vi "All the different Gates.vi"() -> ()   [LabVIEW 2021]
panel:
  out "Boolean 3":bool
  in  "Boolean 2":bool
  in  "Boolean":bool
  out "LED(Output) 6":bool
  in  "B 6":bool
  in  "A 6":bool
  out "LED(Output) 5":bool
  in  "B 5":bool
  in  "A 5":bool
  out "LED(Output) 4":bool
  in  "B 4":bool
  in  "A 4":bool
  out "LED(Output) 3":bool
  in  "B 3":bool
  in  "A 3":bool
  out "LED(Output) 2":bool
  in  "A 2":bool
  out "LED(Output)":bool
  in  "B":bool
  in  "A":bool
  out "LED(Output)":bool
  in  "B":bool
  in  "A":bool
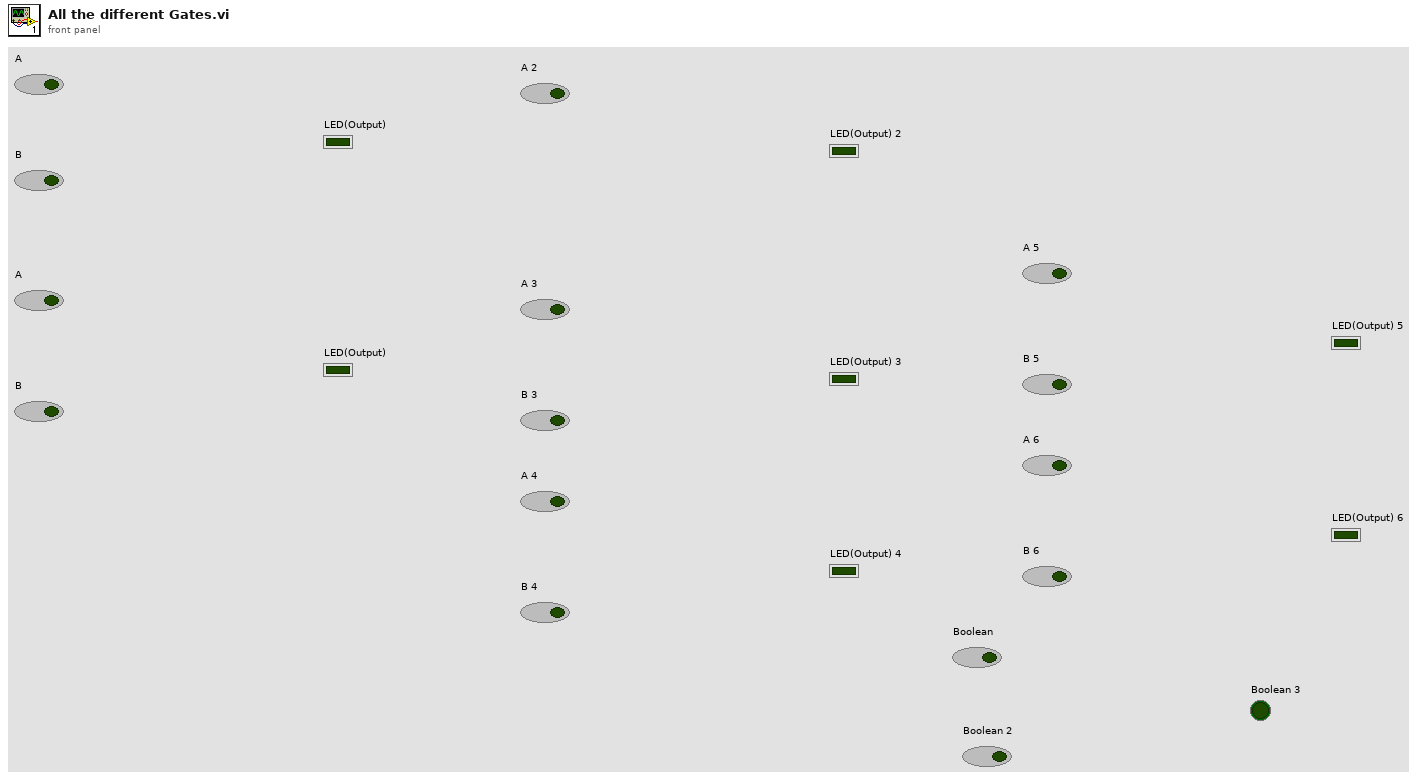
[diagram p1: front panel]
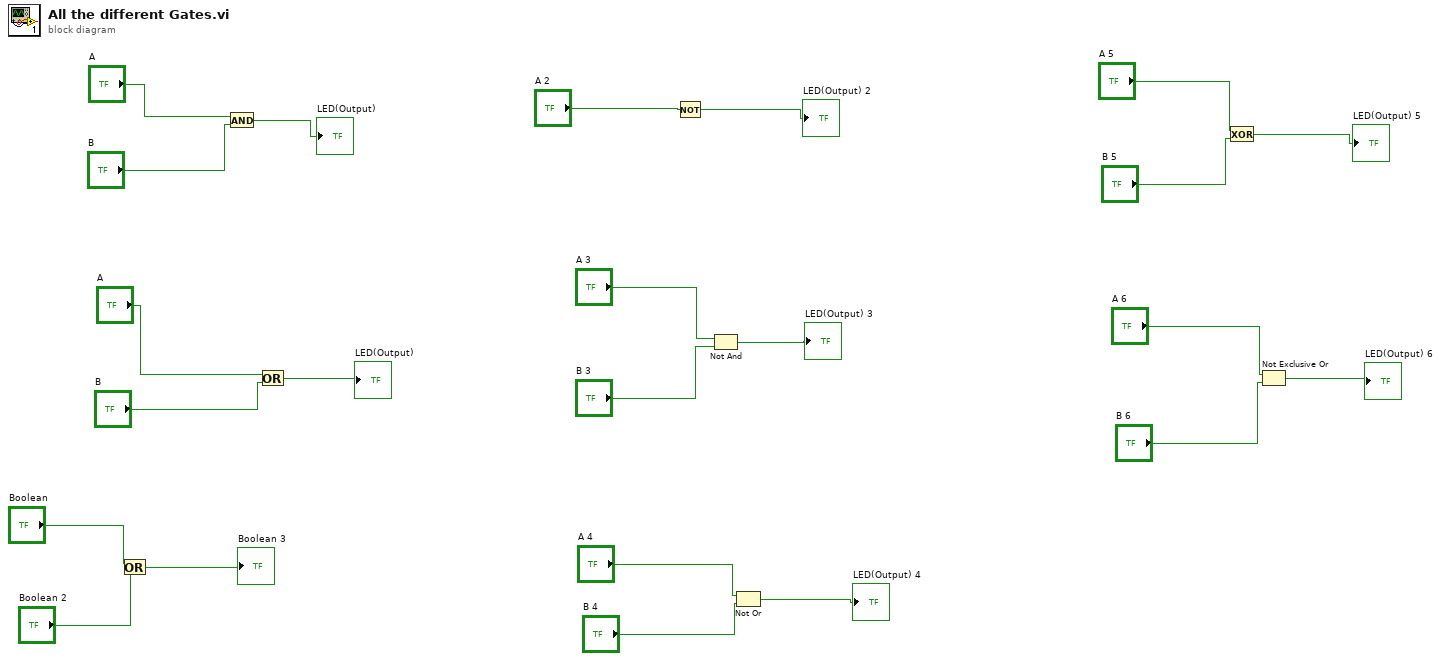
[diagram p0: block diagram]
diagram:
  n1 = Or(x="Boolean", y="Boolean 2") -> (x .or. y?=→"Boolean 3":bool)
  n2 = And(x="A", y="B") -> (x .and. y?=→"LED(Output)":bool)
  n3 = Or(x="A", y="B") -> (x .or. y?=→"LED(Output)":bool)
  n4 = Not(x="A 2") -> (.not. x?=→"LED(Output) 2":bool)
  n5 = Not And(1:"B 3", 2:"A 3") -> (0:→"LED(Output) 3":bool)
  n6 = Not Or(1:"B 4", 2:"A 4") -> (0:→"LED(Output) 4":bool)
  n7 = Exclusive Or(1:"B 5", 2:"A 5") -> (0:→"LED(Output) 5":bool)
  n8 = Not Exclusive Or(1:"B 6", 2:"A 6") -> (0:→"LED(Output) 6":bool)
